vi "Stop Core.vi"(10 "final error code":i32, 11 "IMAQ Display in":refnum<class "HIJ IMAQdx Display.lvclass">) -> (3 "IMAQ Display out":refnum<class "HIJ IMAQdx Display.lvclass">)   [LabVIEW 2014, in "HIJ IMAQdx Display.lvlib" / "HIJ IMAQdx Display.lvclass"]
doc: "(<B>Filename</B>: Actor Framework.lvlib:Actor.lvclass:Stop Core.vi)\n\nDefines what the actor does before it stops. Use the <B>final error code</B> input to determine whether the actor shut down in response to an error.\n\nBy default, this method does nothing. A descendant class may override it to define behavior, such as shutting down any processes the actor initiated in its override of the Actor Core method."
uses:
  HIJ IMAQdx Display.lvclass
  HIJ IMAQdx Display.lvclass/HIJ IMAQdx Display.ctl
  HIJ Vision Display/HIJ Vision Display/HIJ Vision Display.lvclass
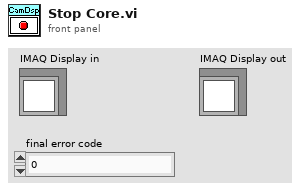
[diagram p1: front panel]
types:
  T1 = typedef "IMAQ Image.ctl" = refnum<image>
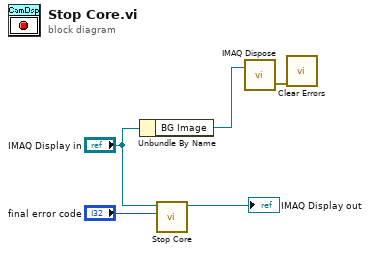
[diagram p0: block diagram]
diagram:
  n1 = Unbundle By Name("IMAQ Display in") -> ("BG Image"=w2:T1)
  n2 = call-parent "Stop Core.vi"("final error code"="final error code", "IMAQ Display in"="IMAQ Display in") -> ("IMAQ Display out"=→"IMAQ Display out":refnum<class "HIJ IMAQdx Display.lvclass">)  [unwired: 9 in]
  n3 = call "IMAQ Dispose"("Image"=w2) -> ("error out"=w1:errorcluster)  [unwired: 5 in]
  n4 = call <vilib>:"Clear Errors.vi"("error in (no error)"=w1) -> ()  [unwired: 5 in, 2 out]
